vi "读配置文件全局2.vi"() -> ()   [LabVIEW 2013]
panel:
  out "加热控制参数判定":bool
  out "充电参数判定":bool
  out "车牌号判定":bool
  out "SOC判定":bool
  out "充电次数时间判定":bool
  out "充放电安时判定":bool
  out "电池包序号判定":bool
  out "电池包信息1判定":bool
  out "三级故障判定":bool
  out "二级故障判定":bool
  out "一级故障判定":bool
  out "温度起始值判定":bool
  out "保险位置判定":bool
  out "通道电压判定":bool
  out "电压起始值判定":bool
  out "从板号判定":bool
  in  "电池组信息":T1
  out "三级故障阀值":dbl[](array[numeric])
  out "二级故障阀值":dbl[](array[numeric])
  out "一级故障阀值":dbl[](array[numeric])
  out "加热控制参数":dbl[](array[numeric])
  out "从板板号":dbl
  in  "表格":string[](array[string])
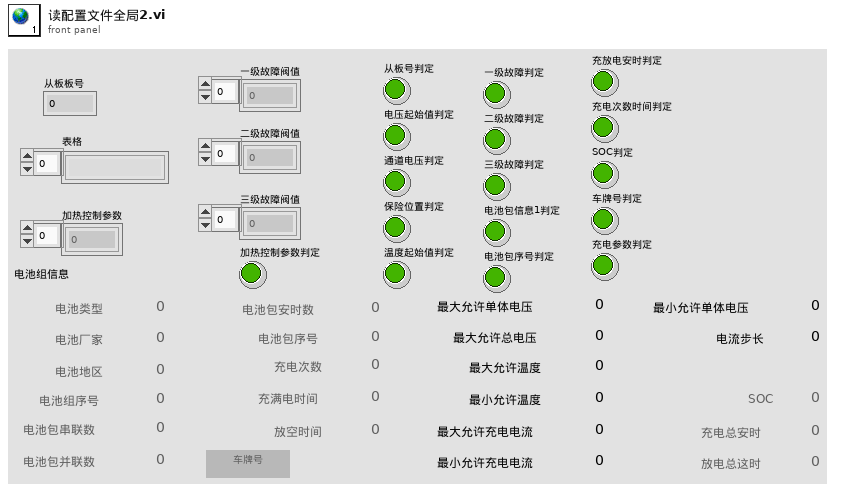
[diagram p1: front panel]
types:
  T1 = cluster{"电池类型":dbl, "电池厂家":dbl, "电池地区":dbl, "电池组序号":dbl, "电池包串联数":dbl, "电池包并联数":dbl, "电池包安时数":dbl, "电池包序号":dbl, "充电次数":dbl, "充满电时间":dbl, "放空时间":dbl, "车牌号":string, "最大允许单体电压":dbl, "最大允许总电压":dbl, "最大允许温度":dbl, "最小允许温度":dbl, "最大允许充电电流":dbl, "最小允许充电电流":dbl, "最小允许单体电压":dbl, "电流步长":dbl, "SOC":dbl, "充电总安时":dbl, "放电总这时":dbl}
diagram:
